vi "Compute BScan.vi"(10 "A-Scan":u32=398, 11 "Array":u16[][](array[numeric])) -> ()   [LabVIEW 2014]
uses:
  <vilib>/Analysis/4window.llb/Hanning Window (DBL).vi
  <vilib>/Analysis/2dsp.llb/Real FFT.vi
  <vilib>/Analysis/4window.llb/AllCosWindow (DBL).vi
  <vilib>/Analysis/NI_AALPro.lvlib
panel:
  out "Intensity Graph":dbl[][](graph)
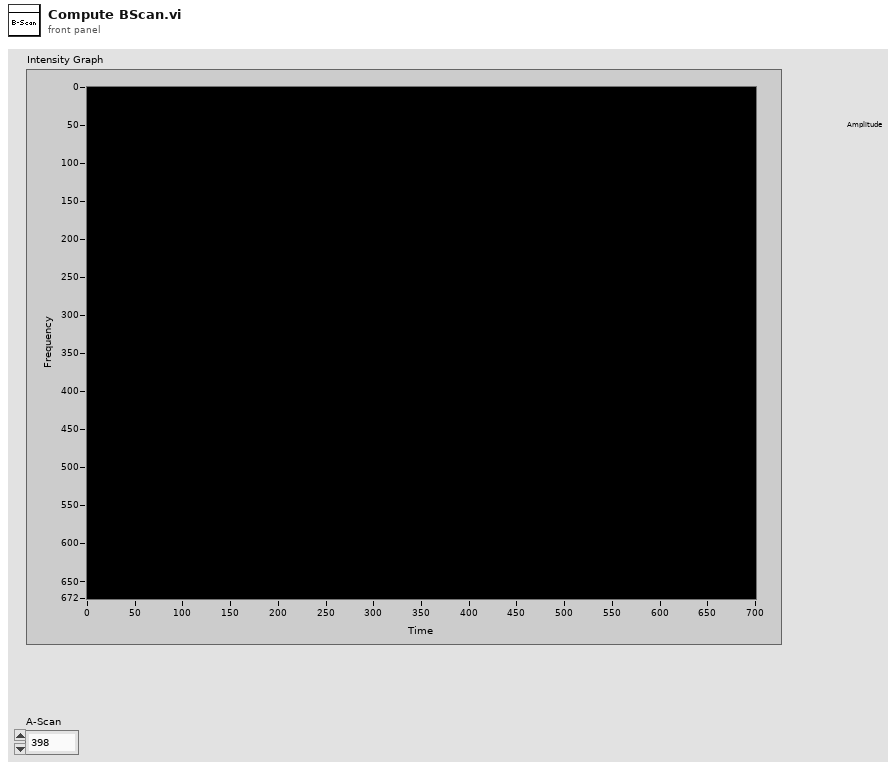
[diagram p1: front panel]
types:
  T1 = typedef "LVCursorListTypeDef.ctl" = cluster{"Name":string, "Color":u32, "Style":u8, "Point Style":u8, "Name Visible":bool, "Allow Drag":bool, "Cursor Mode":u32, "Plot":i32, "Index":i32, "Position":cluster{"X":dbl, "Y":dbl}, "X Scale":u32, "Y Scale":u32, "Watch Plots":i32[], "Watch All Plots":bool, "Plot Area":i32, "Label Offset":cluster{"X":dbl, "Y":dbl}}[]
  T2 = cluster{"Name":string, "Color":u32, "Style":u8, "Point Style":u8, "Name Visible":bool, "Allow Drag":bool, "Cursor Mode":u32, "Plot":i32, "Index":i32, "Position":cluster{"X":dbl, "Y":dbl}, "X Scale":u32, "Y Scale":u32, "Watch Plots":i32[], "Watch All Plots":bool, "Plot Area":i32, "Label Offset":cluster{"X":dbl, "Y":dbl}}
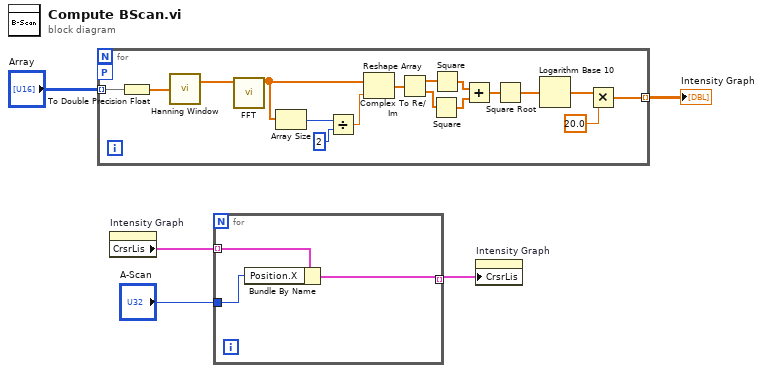
[diagram p0: block diagram]
diagram:
  n1 = for {
    tunnel: "Array" -> [w22] mode=indexing
    workers-P: _ -> [_]
    tunnel: [w6] -> w4 mode=indexing
    n2 = To Double Precision Float(number=w22) -> (double precision float=w21:dbl[])
    n3 = call-poly <vilib>:"Hanning Window.vi"("X"=w21) -> ("Windowed X"=w20:dbl[])  [unwired: 1 out]
    n4 = call-poly <vilib>:"FFT.vi"("X"=w20) -> ("FFT {X}"=w17:cdb[])  [unwired: 9 in, 1 out]
    n5 = Array Size(array=w17) -> (size(s)=w19:i32)
    n6 = Divide(x=w19, y=2) -> (x/y=w16:dbl)
    n7 = Reshape Array(w17, w16) -> (w15:cdb[])
    n8 = Complex To Re/Im(x + iy=w15) -> (x=w14:dbl[], y=w13:dbl[])
    n9 = Square(x=w13) -> (x^2=w11:dbl[])
    n10 = Square(x=w14) -> (x^2=w12:dbl[])
    n11 = Add(x=w12, y=w11) -> (x+y=w10:dbl[])
    n12 = Square Root(x=w10) -> (sqrt(x)=w9:dbl[])
    n13 = Logarithm Base 10(1:w9) -> (0:w8:dbl[])
    n14 = Multiply(x=w8, y=20.0) -> (x*y=w6:dbl[])
  }
  "Intensity Graph" <- w4
  n15 = property on="Intensity Graph" class="IntGraph (strict)"() -> ("CrsrLis"=w3:T1)  [unwired: 2 in, 2 out]
  n16 = for {
    tunnel: w3 -> [w25] mode=indexing
    tunnel: "A-Scan" -> [w24]
    tunnel: [w23] -> w1 mode=indexing
    n17 = Bundle By Name(cluster=w25, "Position.X"=w24) -> (w23:T2)
  }
  n18 = property on="Intensity Graph" class="IntGraph (strict)"("CrsrLis"=w1) -> ()  [unwired: 2 in, 2 out]
